vi "g_VIServerPort.vi"() -> ()   [LabVIEW 2024]
panel:
  in  "Relative VI Path":string="CML.exe\\Libraries\\CML UI\\Main.vi"
  in  "ViServer port number":u16=3355
  # "#EXEs\nNote: For this application independantly communicate with another COM port over another HTTP Port Webservice Port and VI server interface, \n1, Update this Front Panel control, and Right Click - data operations, MAKE CURRENT VALUE DEFAULT, Save.\n2. Update Build Specifications>Web Services? Applications Web Server HTTP Port....This basically just updates the niembeddedws.conf file next to the .exe file\nEXE0 VISERVER: 3350    HTTP: 8002\nEXE1 VISERVER: 3351    HTTP: 8003\nEXE2 VISERVER: 3352    HTTP: 8004\nEXE3 VISERVER: 3353    HTTP: 8005\n3. Update MyComputer>VI Server Port to match this port\n4. Build"
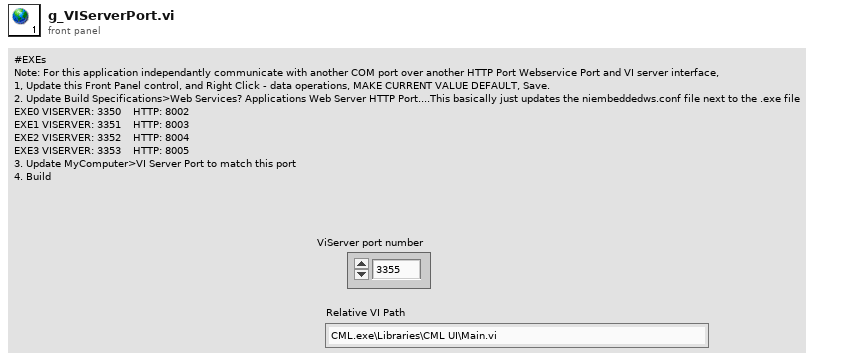
[diagram p1: front panel]
diagram:
